vi "DATA SIMULATION.vi"(7 "Smoothness":dbl, 8 "error in (no error)":errorcluster, 9 "PrevVal":dbl, 10 "MAX":dbl, 11 "MIN":dbl) -> (0 "error out":errorcluster, 3 "Value":dbl)   [LabVIEW 2025]
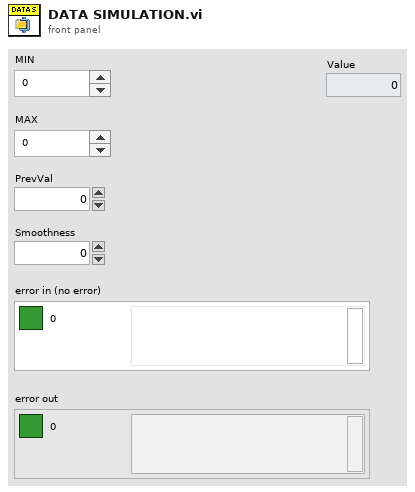
[diagram p1: front panel]
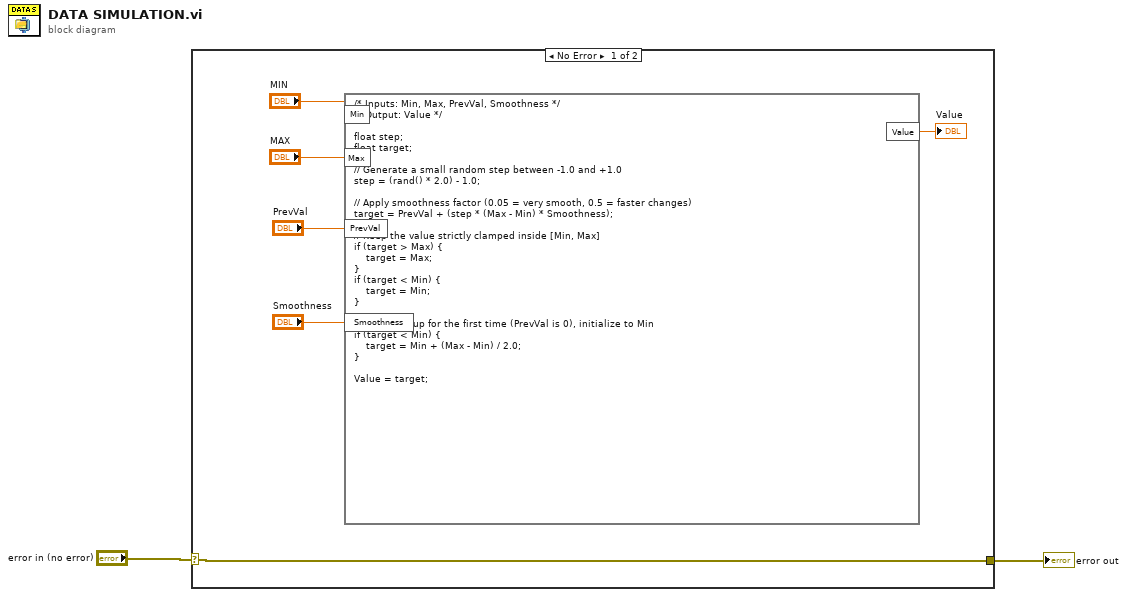
[diagram p0: block diagram]
diagram:
  n1 = case shown="No Error" "error in (no error)" {
    selector: "error in (no error)" -> [w3 _]
    tunnel: [w3 _] -> w1
    frame No Error {
      n2 = formula code="/* Inputs: Min, Max, PrevVal, Smoothness */\n/* Output: Value */\n\nfloat step;\nfloat target;\n\n// Generate a small random step between -1.0 and +1.0\nstep = (rand() * 2.0) - 1.0;\n\n// Apply smoothness factor (0.05 = very smooth, 0.5 = faster changes)\ntarget = PrevVal + (step * (Max - Min) * Smoothness);\n\n// Keep the value strictly clamped inside [Min, Max]\nif (target > Max) {\n    target = Max;\n}\nif (target < Min) {\n    target = Min;\n}\n\n// If starting up for the first time (PrevVal is 0), initialize to Min\nif (target < Min) {\n    target = Min + (Max - Min) / 2.0;\n}\n\nValue = target;"("Min"="MIN", "Max"="MAX", "PrevVal"="PrevVal", "Smoothness"="Smoothness") -> ("Value"=→"Value":dbl)
    }
    frame Error {
    }
  }
  "error out" <- w1
